vi "CTRE_Phoenix_CANcoder_Open.vi"(8 "error in":errorcluster, 10 "Device Number":u8, 11 "CAN Bus":string) -> (0 "error out":errorcluster, 3 "CTRE_CANcoder_DeviceRef":T1)   [LabVIEW 2020]
doc: "Opens a CTRE CANcoder for the given <b>Device Number</b> on the given <b>CAN Bus</b>.\n\n<b>Device Number</b> can be 0 to 63.\n<b>CAN Bus</b> is the string name of the bus. Defaults to empty string which will select the roboRIO's native CAN Bus."
uses:
  <vilib>/Rock Robotics/WPI/ThirdParty/Phoenix-LabVIEW/CANCoder/Controls/CTRE_Phoenix_CANcoder_DeviceRef.ctl
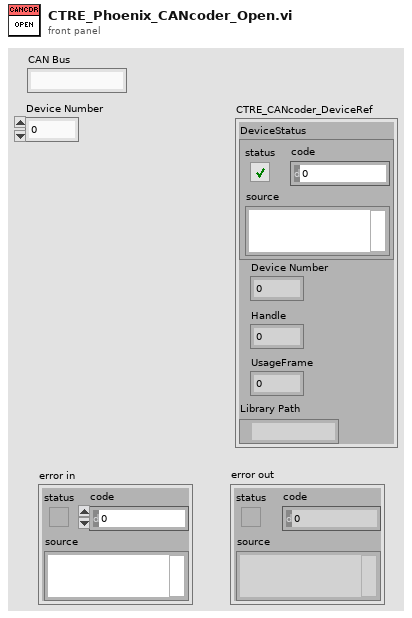
[diagram p1: front panel]
types:
  T1 = typedef "CTRE_Phoenix_CANcoder_DeviceRef.ctl" = cluster{"DeviceStatus":errorcluster, "Device Number":u8, "Handle":u64, "UsageFrame":u32, "Library Path":path}
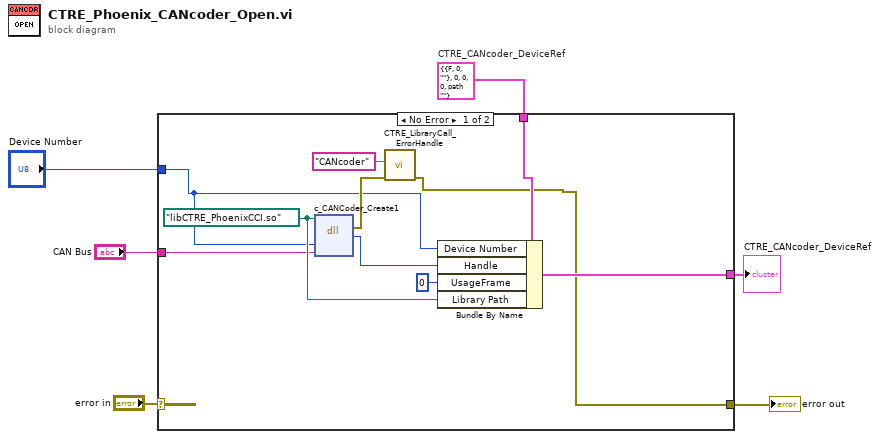
[diagram p0: block diagram]
diagram:
  w3 = T1 {"DeviceStatus"={"status"=FALSE, "code"=0, "source"=""}, "Device Number"=0, "Handle"=0, "UsageFrame"=0, "Library Path"=path ""}  # CTRE_CANcoder_DeviceRef
  n1 = case shown="No Error" "error in" {
    selector: "error in" -> [_ w17]
    tunnel: [w9 w17] -> w5
    tunnel: w3 -> [w16 _]
    tunnel: "Device Number" -> [w8 _]
    tunnel: [w12 _] -> w2
    tunnel: "CAN Bus" -> [w7 _]
    frame No Error {
      w15 = path "libCTRE_PhoenixCCI.so" ("path in")
      n2 = dll-call lib="?" fn="c_CANCoder_Create1"(path in=w15, "deviceNumber"=w8, "canbus"=w7) -> (error out=w11:errorcluster, "handle"=w13:u64)  [unwired: 4 in, 1 out]
      n3 = call <vilib>:"CTRE_LibraryCall_ErrorHandle.vi"("error in"=w11, "DeviceType"="CANcoder") -> ("error out"=w9:errorcluster)  [unwired: 9 in]
      n4 = Bundle By Name(cluster=w16, "Device Number"=w8, "Handle"=w13, "UsageFrame"=u32 0, "Library Path"=w15) -> (w12:T1)
    }
    frame Error {
    }
  }
  "error out" <- w5
  "CTRE_CANcoder_DeviceRef" <- w2
